vi "MakableCheck.vi"(10 "Towels":string[](array[string]), 11 "Pattern":string) -> (3 "Makable":bool)   [LabVIEW 2023, in "2024_19.lvclass"]
uses:
  2024_19.lvclass
  2024_19.lvclass/2024_19.ctl
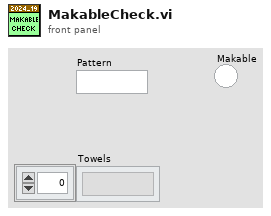
[diagram p1: front panel]
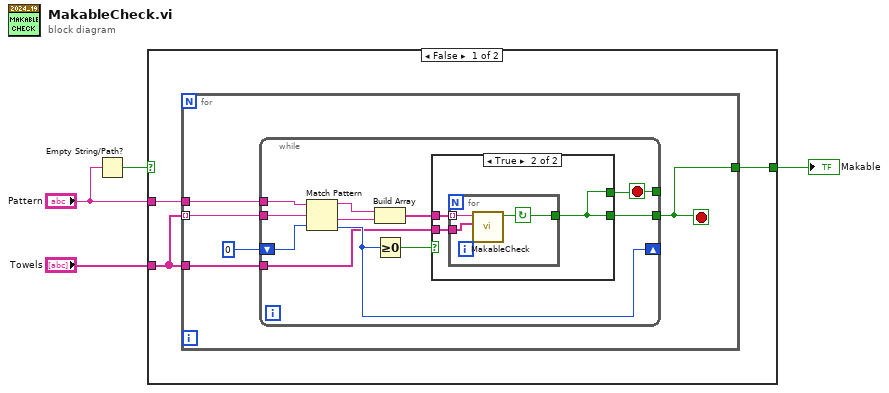
[diagram p0: block diagram]
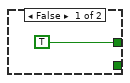
[diagram p2: hidden frame]
diagram:
  n1 = Empty String/Path?(string/path="Pattern") -> (empty?=w2:bool)
  n2 = case shown="False" w2 {
    selector: w2 -> [_ w31]
    tunnel: "Pattern" -> [w7 _]
    tunnel: "Towels" -> [w6 _]
    tunnel: [w5 w31] -> w1
    frame False {
      n3 = for {
        tunnel: w6 -> [w12] mode=indexing
        tunnel: w7 -> [w11]
        tunnel: w6 -> [w9]
        tunnel: [w8] -> w5
        stop <- w8 stop-if-true
        n4 = while {
          tunnel: w12 -> [w21]
          tunnel: w11 -> [w22]
          shift-right: [w20] -> _
          shift-left: 0 -> [w23]
          tunnel: w9 -> [w16]
          tunnel: [w14] -> w8
          tunnel: [w13] -> _
          stop <- w13 stop-if-true
          n5 = Match Pattern(string=w22, regular expression=w21, offset (0)=w23) -> (before substring=w19:string, after substring=w18:string, offset past match=w20:i32)  [unwired: 1 out]
          n6 = Build Array(w19, w18) -> (w17:string[])
          n7 = Greater Or Equal To 0?(x=w20) -> (x >= 0?=w15:bool)
          n8 = case shown="True" w15 {
            tunnel: w17 -> [_ w27]
            tunnel: w16 -> [_ w26]
            tunnel: [_ w25] -> w14
            tunnel: [TRUE ("Makable") w25] -> w13
            frame False {
            }
            frame True {
              n9 = for {
                tunnel: w27 -> [w30] mode=indexing
                tunnel: w26 -> [w29]
                tunnel: [w28] -> w25
                stop <- w28 continue-if-true
                n10 = call "MakableCheck.vi"("Towels"=w29, "Pattern"=w30) -> ("Makable"=w28:bool)  [unwired: 9 in]
              }
            }
          }
        }
      }
    }
    frame True {
    }
  }
  "Makable" <- w1
